vi "sendAndReadTelemetry.vi"(6 "telFrecuencyInHz (10)":u32=100, 8 "error in (no error)":errorcluster, 9 "numPackets (50)":i32=50, 10 "tel connection in":refnum<k5>, 11 "TcpServer out":refnum<class "TcpServer.lvclass">) -> (0 "error out":errorcluster, 1 "telemetry received":string[](array[string]), 2 "tel connection out":refnum<k5>, 3 "tcpServer out":refnum<class "TcpServer.lvclass">)   [LabVIEW 2018]
doc: "Generate elements defined by the numPackets control and send them as telemetry to TCP client, at a rate defined by the telFrecuencyInHz control. Then, read them. The default value of number of packets is 50, and the frecuency rate is 10 Hz."
uses:
  src/TcpServer/TcpServer.lvclass
  src/TcpServerTel/typedef/telTypeDef.ctl
  src/TcpServerTel/TcpServerTel.lvclass
panel:
  out "rate (Hz)":dbl format="%#_4f"
  out "time (sec)":dbl
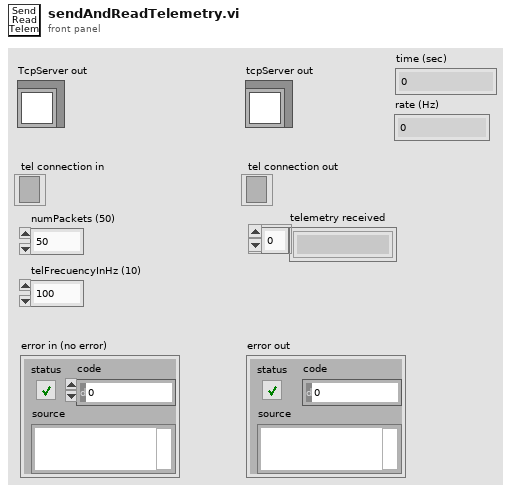
[diagram p1: front panel]
types:
  T1 = typedef "TcpServerTel.lvclass/telTypeDef.ctl" = cluster{"name":string, "telDetails":string}
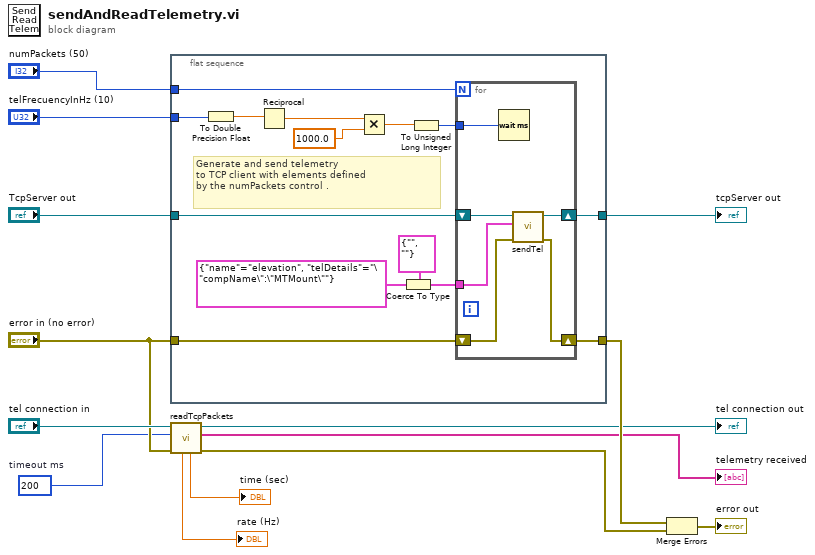
[diagram p0: block diagram]
diagram:
  w5 = 200  # timeout ms
  n1 = flat-sequence {
    tunnel: "TcpServer out" -> [w28]
    tunnel: "error in (no error)" -> [w27]
    tunnel: [w26] -> w12
    tunnel: [w22] -> w13
    tunnel: "numPackets (50)" -> [w21]
    tunnel: "telFrecuencyInHz (10)" -> [w20]
    frame #0 {
      # "Generate and send telemetry\nto TCP client with elements defined\nby the numPackets control ."
      n2 = To Double Precision Float(number=w20) -> (double precision float=w19:dbl)
      n3 = Reciprocal(x=w19) -> (1/x=w18:dbl)
      n4 = Multiply(x=w18, y=1000.0) -> (x*y=w16:dbl)
      n5 = Coerce To Type(0:T1 {"name"="elevation", "telDetails"="\"compName\":\"MTMount\""} ("x"), 1:T1 {"name"="", "telDetails"=""} ("Telemetry")) -> (2:w24:T1)
      n6 = To Unsigned Long Integer(number=w16) -> (unsigned 32bit integer=w15:u32)
      n7 = for {
        N: w21 -> [_]
        tunnel: w24 -> [w30]
        shift-right: [w31] -> w22
        shift-left: w28 -> [w33]
        shift-right: [w34] -> w26
        shift-left: w27 -> [w32]
        tunnel: w15 -> [w29]
        n8 = Wait (ms)(milliseconds to wait=w29) -> ()  [unwired: 1 out]
        n9 = call "sendTel.vi"("error in (no error)"=w32, "Telemetry"=w30, "tcpServer in"=w33) -> ("error out"=w34:errorcluster, "tcpServer out"=w31:refnum<class "TcpServer.lvclass">)  [unwired: 7 in]
      }
    }
  }
  n10 = call "readTcpPackets.vi"("error in (no error)"="error in (no error)", "timeout ms"=w5, "connection ID in"="tel connection in") -> ("error out"=w7:errorcluster, "TCP packets"=→"telemetry received":string[], "connection ID out"=→"tel connection out":refnum<k5>, "seconds"=→"time (sec)":dbl, "rate (Hz)"=→"rate (Hz)":dbl)  [unwired: 4 in]
  n11 = Merge Errors(w12, w7) -> (→"error out":errorcluster)
  "tcpServer out" <- w13
